vi "WLAN Tx Test Limits LSL SymbolClock.vi"(8 "error in (no error)":errorcluster, 10 "Limits":T1 {"OBW"."Stop Frequency (Hz)" format="%#_4p"; "OBW"."Start Frequency (Hz)" format="%#_4p"; "OBW"."OBW (Hz)" format="%#_4p"}, 11 "WLAN Tx Test in":refnum<class "niDTS WLAN Tx Test.lvclass">) -> (0 "error out":errorcluster, 2 "Limits Out":T1 {"OBW"."Stop Frequency (Hz)" format="%#_4p"; "OBW"."Start Frequency (Hz)" format="%#_4p"; "OBW"."OBW (Hz)" format="%#_4p"}, 3 "WLAN Tx Test out":refnum<class "niDTS WLAN Tx Test.lvclass">)   [LabVIEW 2015, in "niDTS WLAN.lvlib" / "niDTS WLAN Tx Test.lvclass"]
uses:
  niDTS WLAN Tx Test.lvclass
  Includes/niDTS WLAN Tx Test INC Results.ctl
  Includes/niDTS WLAN Tx Test INC MOD EVM Results.ctl
  Includes/Results/niDTS Tx RES INC EVM.ctl
  Includes/niDTS WLAN Tx Test INC TXP Results.ctl
  Includes/niDTS WLAN Tx Test INC TXP Result SINGLE.ctl
  Includes/niDTS WLAN Tx Test INC OBW Results.ctl
  Instrument/INSTR TX/Results/niDTS WLAN INSTR TX INC SEM Results.ctl
  Instrument/INSTR TX/Results/niDTS WLAN INSTR TX INC SEM FSEGemts Results.ctl
  Includes/Results/niDTS Tx RES INC SEM FSEGemts.ctl
  Instrument/INSTR TX/Results/niDTS WLAN INSTR TX INC SEM MARGin Results.ctl
  Includes/Results/niDTS Tx RES INC SEM Margin.ctl
  Instrument/INSTR TX/Results/niDTS WLAN INSTR TX INC OFDM Impairments Results.ctl
  niDTS WLAN Tx Test.lvclass/niDTS WLAN Tx Test.ctl
  niDTS WLAN.lvlib
  Instrument/INSTR TX/niDTS WLAN INSTR TX.lvclass
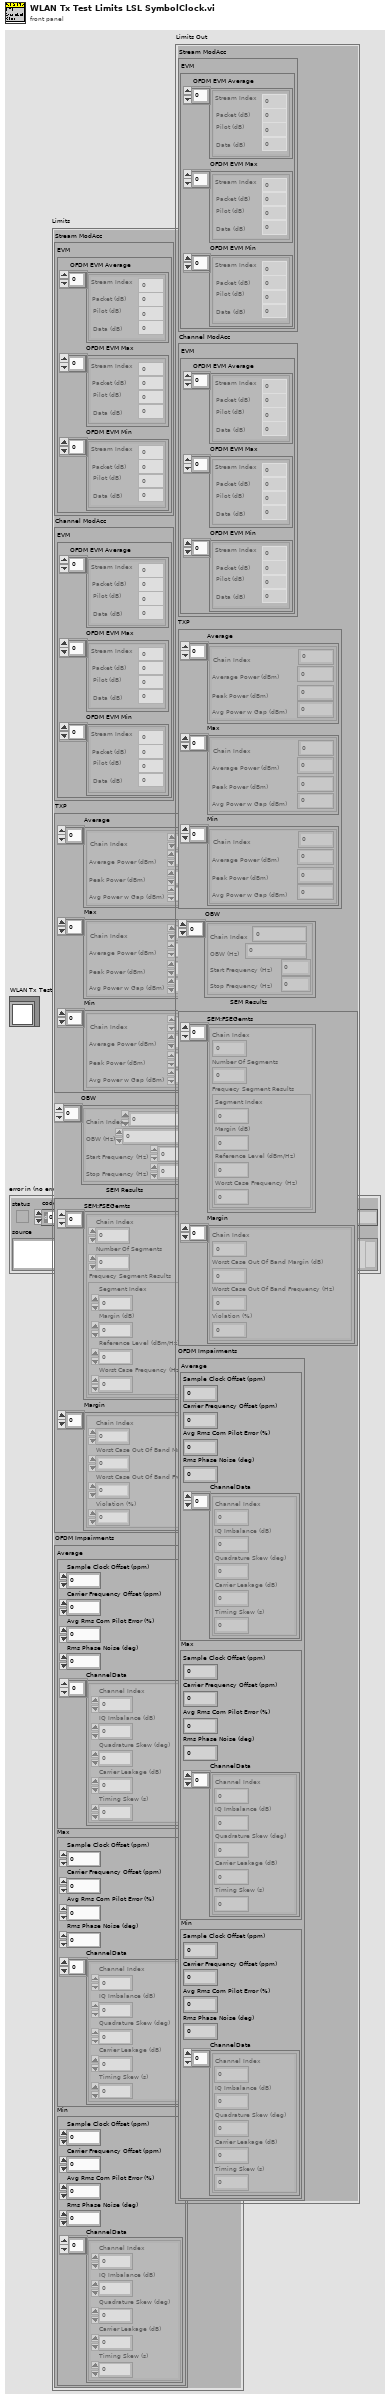
[diagram p1: front panel]
types:
  T1 = typedef "niDTS WLAN.lvlib/niDTS WLAN Tx Test INC Results.ctl" = cluster{"Stream ModAcc":T2, "Channel ModAcc":T2, "TXP":T4, "OBW":T6[], "SEM Results":T7, "OFDM Impairments":T12}
  T2 = typedef "niDTS WLAN.lvlib/niDTS WLAN Tx Test INC MOD EVM Results.ctl" = cluster{"EVM":cluster{"OFDM EVM Average":T3[], "OFDM EVM Max":T3[], "OFDM EVM Min":T3[]}}
  T3 = typedef "niDTS WLAN.lvlib/niDTS Tx RES INC EVM.ctl" = cluster{"Stream Index":i32, "Packet (dB)":dbl, "Pilot (dB)":dbl, "Data (dB)":dbl}
  T4 = typedef "niDTS WLAN.lvlib/niDTS WLAN Tx Test INC TXP Results.ctl" = cluster{"Average":T5[], "Max":T5[], "Min":T5[]}
  T5 = typedef "niDTS WLAN.lvlib/niDTS WLAN Tx Test INC TXP Result SINGLE.ctl" = cluster{"Chain Index":dbl, "Average Power (dBm)":dbl, "Peak Power (dBm)":dbl, "Avg Power w Gap (dBm)":dbl}
  T6 = typedef "niDTS WLAN.lvlib/niDTS WLAN Tx Test INC OBW Results.ctl" = cluster{"Chain Index":dbl, "OBW (Hz)":dbl, "Start Frequency (Hz)":dbl, "Stop Frequency (Hz)":dbl}
  T7 = typedef "niDTS WLAN.lvlib/niDTS WLAN INSTR TX.lvclass/niDTS WLAN INSTR TX INC SEM Results.ctl" = cluster{"SEM:FSEGemts":T8, "Margin":T10}
  T8 = typedef "niDTS WLAN.lvlib/niDTS WLAN INSTR TX.lvclass/niDTS WLAN INSTR TX INC SEM FSEGemts Results.ctl" = T9[]
  T9 = typedef "niDTS WLAN.lvlib/niDTS Tx RES INC SEM FSEGemts.ctl" = cluster{"Chain Index":i32, "Number Of Segments":i32, "Frequecy Segment Results":cluster{"Segment Index":i32, "Margin (dB)":dbl, "Reference Level (dBm/Hz)":dbl, "Worst Case Frequency (Hz)":dbl}}
  T10 = typedef "niDTS WLAN.lvlib/niDTS WLAN INSTR TX.lvclass/niDTS WLAN INSTR TX INC SEM MARGin Results.ctl" = T11[]
  T11 = typedef "niDTS WLAN.lvlib/niDTS Tx RES INC SEM Margin.ctl" = cluster{"Chain Index":i32, "Worst Case Out Of Band Margin (dB)":dbl, "Worst Case Out Of Band Frequency (Hz)":dbl, "Violation (%)":dbl}
  T12 = typedef "niDTS WLAN.lvlib/niDTS WLAN INSTR TX.lvclass/niDTS WLAN INSTR TX INC OFDM Impairments Results.ctl" = cluster{"Average":cluster{"Sample Clock Offset (ppm)":dbl, "Carrier Frequency Offset (ppm)":dbl, "Avg Rms Com Pilot Error (%)":dbl, "Rms Phase Noise (deg)":dbl, "ChannelData":cluster{"Channel Index":i32, "IQ Imbalance (dB)":dbl, "Quadrature Skew (deg)":dbl, "Carrier Leakage (dB)":dbl, "Timing Skew (s)":dbl}[]}, "Max":cluster{"Sample Clock Offset (ppm)":dbl, "Carrier Frequency Offset (ppm)":dbl, "Avg Rms Com Pilot Error (%)":dbl, "Rms Phase Noise (deg)":dbl, "ChannelData":cluster{"Channel Index":i32, "IQ Imbalance (dB)":dbl, "Quadrature Skew (deg)":dbl, "Carrier Leakage (dB)":dbl, "Timing Skew (s)":dbl}[]}, "Min":cluster{"Sample Clock Offset (ppm)":dbl, "Carrier Frequency Offset (ppm)":dbl, "Avg Rms Com Pilot Error (%)":dbl, "Rms Phase Noise (deg)":dbl, "ChannelData":cluster{"Channel Index":i32, "IQ Imbalance (dB)":dbl, "Quadrature Skew (deg)":dbl, "Carrier Leakage (dB)":dbl, "Timing Skew (s)":dbl}[]}}
  T13 = typedef "niDTS WLAN.lvlib/niDTS WLAN INC Standard.ctl" = enum16{"802.11 b DSSS", "802.11 a/g OFDM", "802.11 n HT", "802.11 ac VHT"}
  T14 = typedef "niDTS WLAN.lvlib/niDTS WLAN INC CH BW.ctl" = enum16{"20 MHz", "40 MHz", "80 MHz", "160 MHz"}
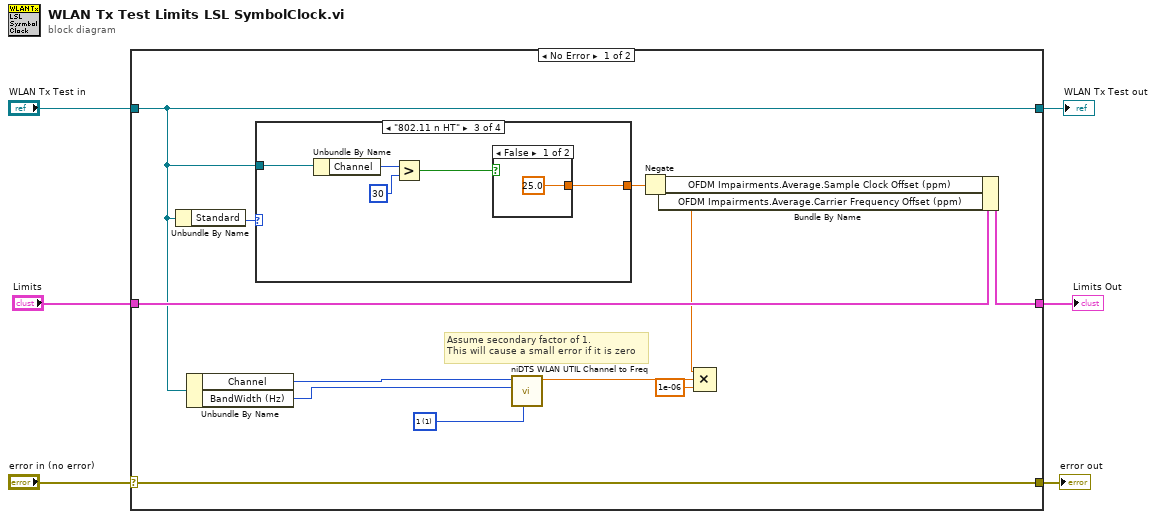
[diagram p0: block diagram]
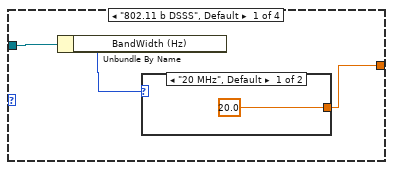
[diagram p2: hidden frame]
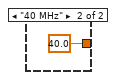
[diagram p3: hidden frame]
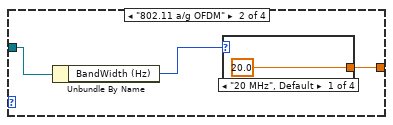
[diagram p4: hidden frame]
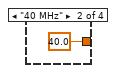
[diagram p5: hidden frame]
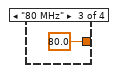
[diagram p6: hidden frame]
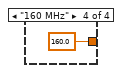
[diagram p7: hidden frame]
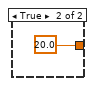
[diagram p8: hidden frame]
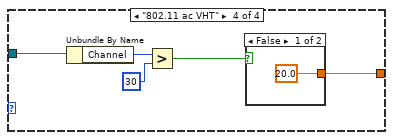
[diagram p9: hidden frame]
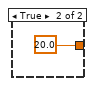
[diagram p10: hidden frame]
diagram:
  n1 = case shown="No Error" "error in (no error)" {
    selector: "error in (no error)" -> [w18 w47]
    tunnel: [w18 w47] -> w5
    tunnel: [w10 w46] -> w3
    tunnel: "WLAN Tx Test in" -> [w10 w46]
    tunnel: "Limits" -> [w16 w45]
    tunnel: [w8 w45] -> w1
    frame No Error {
      w9 = 1 items=["-1"=-1, "1"=1, "0"=0] ("secondary factor")
      # "Assume secondary factor of 1.\nThis will cause a small error if it is zero"
      n2 = Unbundle By Name(w10) -> ("Standard"=w17:T13)
      n3 = Unbundle By Name(w10) -> ("Channel"=w11:i32, "BandWidth (Hz)"=w12:T14)
      n4 = case shown="\"802.11 n HT\"" w17 {
        tunnel: w10 -> [w21 w26 w35 w42]
        tunnel: [w19 w24 w31 w38] -> w15
        frame "802.11 b DSSS", Default {
          n5 = Unbundle By Name(w21) -> ("BandWidth (Hz)"=w20:T14)
          n6 = case shown="\"20 MHz\", Default" w20 {
            tunnel: [20.0 40.0] -> w19
            frame "20 MHz", Default {
            }
            frame "40 MHz" {
            }
          }
        }
        frame "802.11 a/g OFDM" {
          n7 = Unbundle By Name(w26) -> ("BandWidth (Hz)"=w25:T14)
          n8 = case shown="\"20 MHz\", Default" w25 {
            tunnel: [20.0 40.0 80.0 160.0] -> w24
            frame "20 MHz", Default {
            }
            frame "40 MHz" {
            }
            frame "80 MHz" {
            }
            frame "160 MHz" {
            }
          }
        }
        frame "802.11 n HT" {
          n9 = Unbundle By Name(w35) -> ("Channel"=w34:i32)
          n10 = Greater?(x=w34, y=30) -> (0:w32:bool)
          n11 = case shown="False" w32 {
            tunnel: [25.0 20.0] -> w31
            frame False {
            }
            frame True {
            }
          }
        }
        frame "802.11 ac VHT" {
          n12 = Unbundle By Name(w42) -> ("Channel"=w41:i32)
          n13 = Greater?(x=w41, y=30) -> (0:w39:bool)
          n14 = case shown="False" w39 {
            tunnel: [20.0 20.0] -> w38
            frame False {
            }
            frame True {
            }
          }
        }
      }
      n15 = call "niDTS WLAN UTIL Channel to Freq.vi"("secondary factor"=w9, "CH BW"=w12, "Channel"=w11) -> ("Center Frequency (Hz)"=w13:dbl)  [unwired: 6 in, 2 out]
      n16 = Negate(x=w15) -> (-x=w7:dbl)
      n17 = Bundle By Name(cluster=w16, "OFDM Impairments.Average.Sample Clock Offset (ppm)"=w7, "OFDM Impairments.Average.Carrier Frequency Offset (ppm)"=w7) -> (w8:T1)
      n18 = Compound Arithmetic op=MULTIPLY(w7, w13, 1e-06 ("value")) -> ()  [unwired: 1 out]
    }
    frame Error {
    }
  }
  "error out" <- w5
  "WLAN Tx Test out" <- w3
  "Limits Out" <- w1
